vi "SaveDefaultValues.vi"(2 "Step":enum16{"Start", "Save"}(ring)=enum."Save", 5 "VI to save":path=path "C:/Users/chchung/Desktop/project/Door/DoorAccess.vi", 11 "error in (no error)":errorcluster) -> (15 "error out":errorcluster)   [LabVIEW 2011]
doc: "See description in wait.vi"
panel:
  out "appended path":path
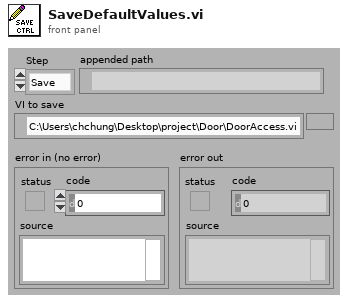
[diagram p1: front panel]
types:
  T1 = typedef "Rendezvous RefNum" = refnum<k1>
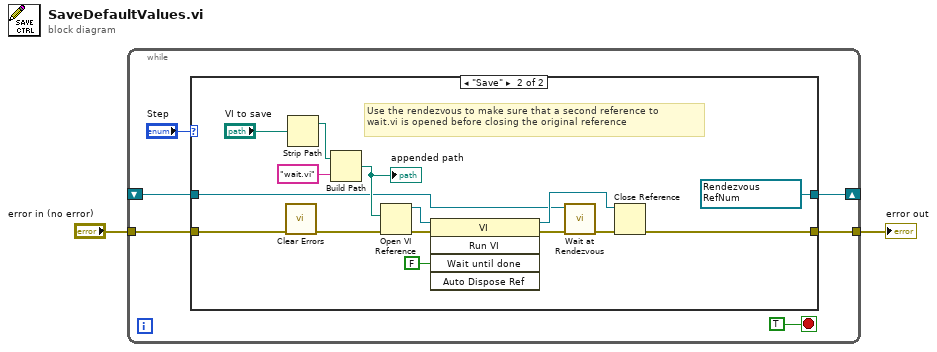
[diagram p0: block diagram]
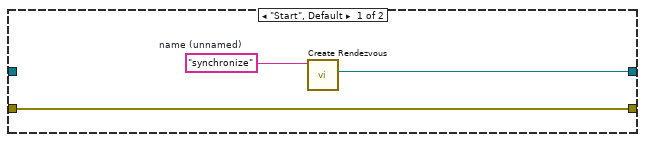
[diagram p2: hidden frame]
diagram:
  n1 = while {
    shift-right: [w7] -> _
    shift-left: _ -> [w5]
    tunnel: "error in (no error)" -> [w4]
    tunnel: [w3] -> w1
    stop <- TRUE stop-if-true
    n2 = case shown="\"Save\"" "Step" {
      tunnel: [w10 w14] -> w7
      tunnel: w5 -> [_ w17]
      tunnel: w4 -> [w9 w13]
      tunnel: [w9 w15] -> w3
      frame "Start", Default {
        w11 = "synchronize"  # name (unnamed)
        n3 = call <vilib>:"Create Rendezvous.vi"("name (unnamed)"=w11) -> ("rendezvous"=w10:T1)  [unwired: 4 in, 2 out]
      }
      frame "Save" {
        w14 = T1 refnum items=["rendezvous"] ("rendezvous")
        # "Use the rendezvous to make sure that a second reference to \nwait.vi is opened before closing the original reference"
        n4 = call <vilib>:"Clear Errors.vi"("error in (no error)"=w13) -> ("error out"=w12:errorcluster)  [unwired: 6 in]
        n5 = Strip Path(path="VI to save") -> (stripped path=w20:path)  [unwired: 1 out]
        n6 = Build Path(base path=w20, name or relative path="wait.vi") -> (appended path=w18:path)
        "appended path" <- w18
        n7 = Open VI Reference(vi path=w18, error in (no error)=w12) -> (vi reference=w25:refnum<vi>, error out=w24:errorcluster)  [unwired: 4 in]
        n8 = invoke class="VI" method="Run VI"(reference=w25, error in=w24, "Wait until done"=FALSE) -> (reference out=w23:refnum<vi>, error out=w22:errorcluster)  [unwired: 2 in, 3 out]
        n9 = call <vilib>:"Wait at Rendezvous.vi"("error in (no error)"=w22, "rendezvous"=w17) -> ("error out"=w21:errorcluster)  [unwired: 3 in, 2 out]
        n10 = Close Reference(reference=w23, error in (no error)=w21) -> (error out=w15:errorcluster)
      }
    }
  }
  "error out" <- w1
